vi "Generate pulse.vi"(10 "Pulse magnitude":dbl, 11 "Waveform parameters":T1={"Start magnitude"=0.0, "Magnitude increment"=0.0, "Number of pulses"=0, "Ramp length"=0, "Top  length"=0, "Threshold "=3000, "Processing delay"=240, "Stop after"=1, "Detector window"=480} {"Detector window" format="%dpts"; "Stop after" format="%d sweep(s)"}) -> (2 "Data out":dbl[](array[numeric]), 3 "Waveform parameters out":T1={"Start magnitude"=0.0, "Magnitude increment"=0.0, "Number of pulses"=0, "Ramp length"=0, "Top  length"=0, "Threshold "=3000, "Processing delay"=240, "Stop after"=1, "Detector window"=480} {"Detector window" format="%dpts"; "Stop after" format="%d sweep(s)"})   [LabVIEW 2016]
uses:
  Waveform parameters.ctl
panel:
  out "Waveform Graph":dbl[](graph)
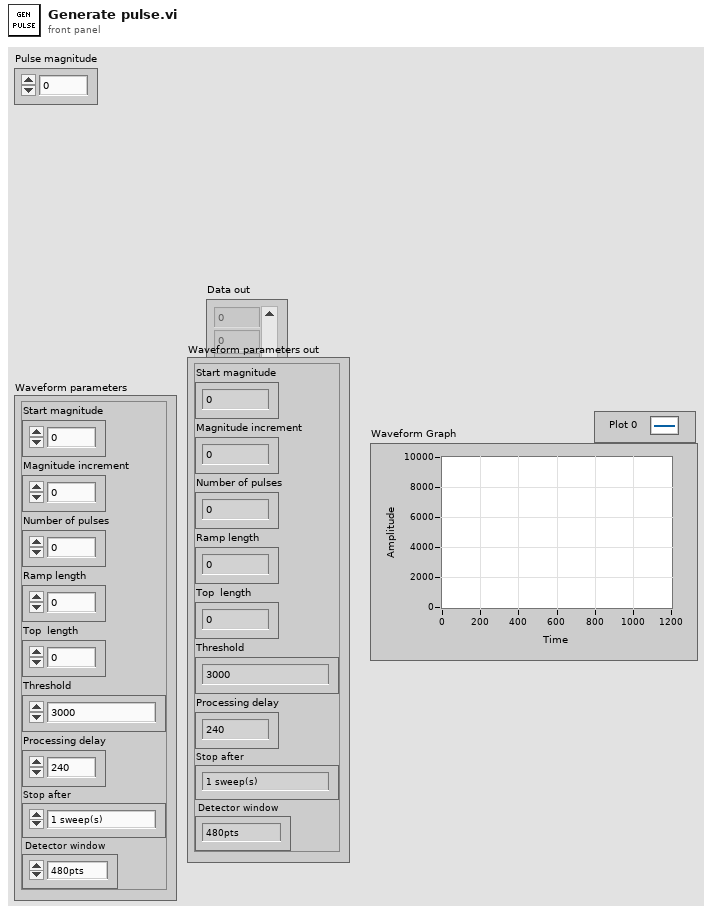
[diagram p1: front panel]
types:
  T1 = typedef "Waveform parameters.ctl" = cluster{"Start magnitude":dbl, "Magnitude increment":dbl, "Number of pulses":i32, "Ramp length":i32, "Top  length":i32, "Threshold ":i32, "Processing delay":u16, "Stop after":u16, "Detector window":i32}
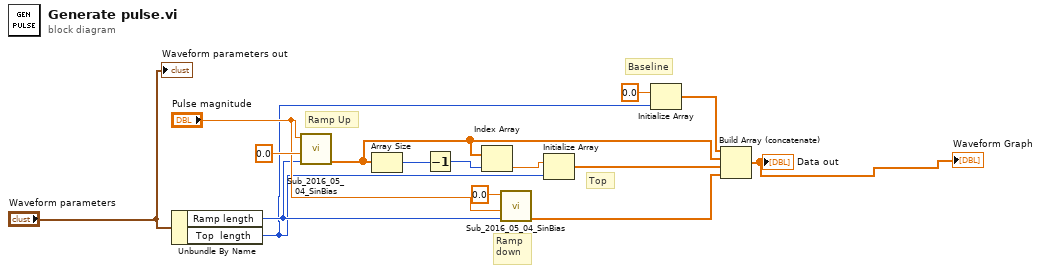
[diagram p0: block diagram]
diagram:
  # "Baseline"
  # "Ramp Up"
  # "Ramp \ndown"
  # "Top"
  n1 = Unbundle By Name("Waveform parameters") -> ("Ramp length"=w4:i32, "Top  length"=w1:i32)
  n2 = call "Sub_2016_05_04_SinBias.vi"("Number of steps"=w4, "Start current"=0.0, "Finish current"="Pulse magnitude") -> ("Array 2"=w7:dbl[])  [unwired: 7 in, 1 out]
  n3 = Array Size(array=w7) -> (size(s)=w6:i32)
  n4 = Decrement(x=w6) -> (x-1=w14:i32)
  n5 = Index Array(array=w7, index=w14) -> (element=w11:dbl)
  n6 = call "Sub_2016_05_04_SinBias.vi"("Number of steps"=w4, "Start current"="Pulse magnitude", "Finish current"=0.0) -> ("Array 2"=w8:dbl[])  [unwired: 7 in, 1 out]
  n7 = Initialize Array(w11, w1) -> (w9:dbl[])
  n8 = Initialize Array(0.0, w1) -> (w10:dbl[])
  n9 = Build Array (concatenate)(w10, w7, w9, w8) -> (→"Data out" →"Waveform Graph":dbl[])
  "Waveform parameters out" <- "Waveform parameters"
